vi "Config - Interface.vi"(8 "error in (no error)":errorcluster, 11 "View Model":T1) -> (0 "error out":errorcluster, 3 "View Model":T1)   [LabVIEW 2017]
doc: "A separate user interface of configuration process.\n[Covers: SD6]"
uses:
  Controls/Config Record.ctl
  View Model/Controls/View Model.ctl
  View Model/Controls/Shared Model.ctl
  Error Handler/Controls/Error Model.ctl
  Error Handler/Controls/Error Data.ctl
  Error Handler/Controls/Error Level.ctl
  Controls/Config Model.ctl
  Controls/Config Data.ctl
  Controls/Config Command.ctl
panel:
  in  "Update":bool
  in  "Insert":bool
  in  "Query":bool
  in  "Read":bool
  in  "Current Configuration Database":T5[](array[typedef])
  in  "Config Record (Insert/Update)":T5
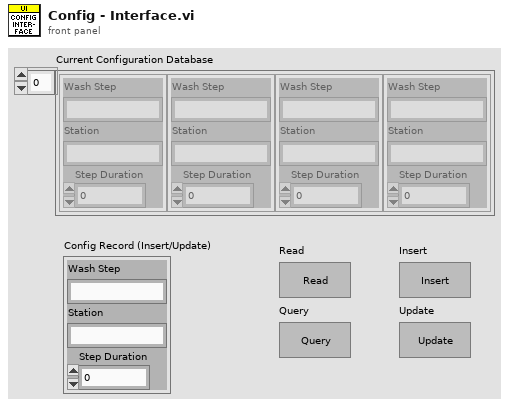
[diagram p1: front panel]
types:
  T1 = typedef "View Model.ctl" = cluster{"Shared Model":T2, "Error Model":T3, "Config Model":T4}
  T2 = typedef "Shared Model.ctl" = cluster{"Stop":refnum<user-event>, "Stop DVR":refnum<data-value>}
  T3 = typedef "Error Model.ctl" = cluster{"Error":refnum<user-event>}
  T4 = typedef "Config Model.ctl" = cluster{"Config Recs DVR":refnum<data-value>, "Config Data":refnum<user-event>, "Config Lock":refnum<user-event>, "Config Lock DVR":refnum<data-value>}
  T5 = typedef "Config Record.ctl" = cluster{"Wash Step":string, "Station":string, "Step Duration":u32}
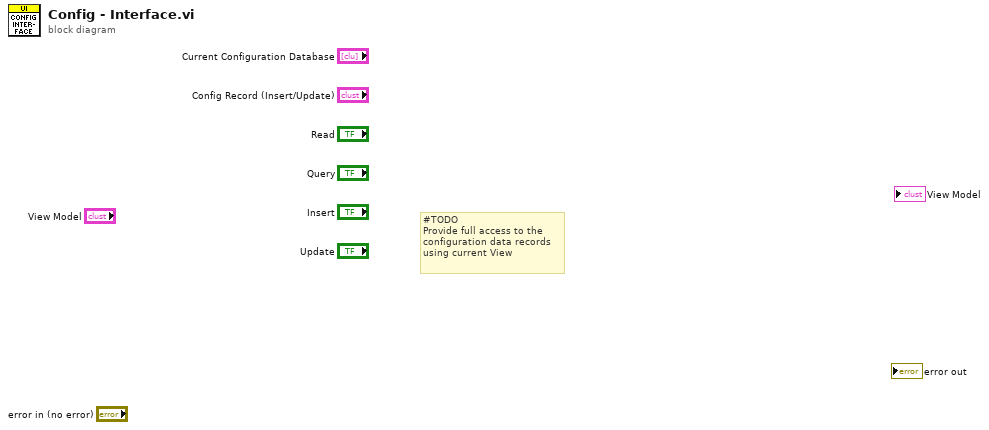
[diagram p0: block diagram]
diagram:
  # "#TODO\nProvide full access to the \nconfiguration data records\nusing current View"
